vi "Enqueue Message.vi"(7 "Priority Message":bool, 8 "error in (no error)":errorcluster, 9 "Message Data":variant, 10 "Message":string, 11 "Queue in":refnum<queue>) -> (0 "error out":errorcluster, 3 "Queue out":refnum<queue>)   [LabVIEW 2014]
uses:
  Controls/Message Cluster.ctl
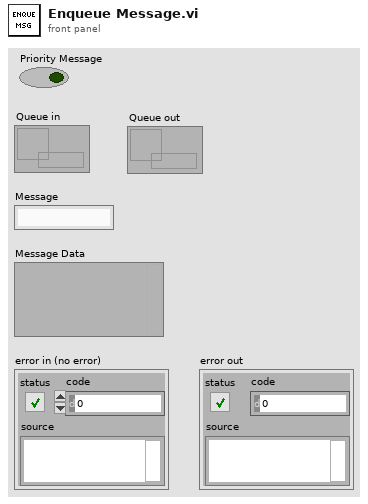
[diagram p1: front panel]
types:
  T1 = typedef "Message Cluster.ctl" = cluster{"Message":string, "Message Data":variant}
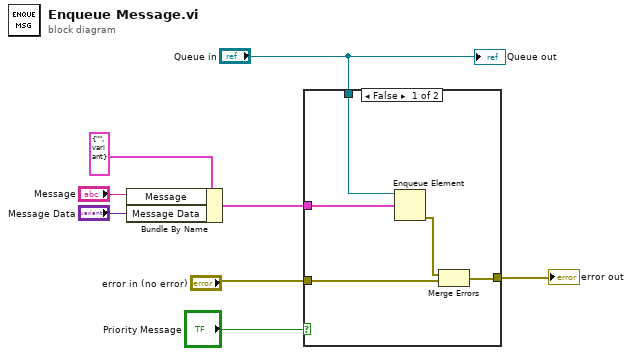
[diagram p0: block diagram]
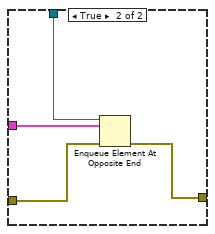
[diagram p2: hidden frame]
diagram:
  n1 = Bundle By Name(cluster=T1 {"Message"="", "Message Data"=variant} ("Message Cluster"), "Message"="Message", "Message Data"="Message Data") -> (w5:T1)
  n2 = case shown="False" "Priority Message" {
    tunnel: w5 -> [w13 w17]
    tunnel: [w9 w15] -> w7
    tunnel: "error in (no error)" -> [w10 w16]
    tunnel: "Queue in" -> [w12 w14]
    frame False {
      n3 = Enqueue Element(queue=w12, element=w13) -> (error out=w11:errorcluster)  [unwired: 2 in, 2 out]
      n4 = Merge Errors(w11, w10) -> (w9:errorcluster)
    }
    frame True {
      n5 = Enqueue Element At Opposite End(queue=w14, element=w17, error in (no error)=w16) -> (error out=w15:errorcluster)  [unwired: 1 in, 2 out]
    }
  }
  "error out" <- w7
  "Queue out" <- "Queue in"
